vi "Register Message Metadata.vi"(8 "error in":errorcluster, 10 "Messages":T2[](array[typedef]), 11 "gRPCid in":T1) -> (0 "error out":errorcluster, 3 "gRPCid out":T1)   [LabVIEW 2019, in "grpc-lvsupport.lvlib"]
uses:
  grpc-lvsupport.lvlib
  typeDefs/Message Metadata.ctl
  typeDefs/Message Element Metadata.ctl
  typeDefs/Message Element Type.ctl
  Shared/grpcId.ctl
  <vilib>/Utility/error.llb/Error Cluster From Error Code.vi
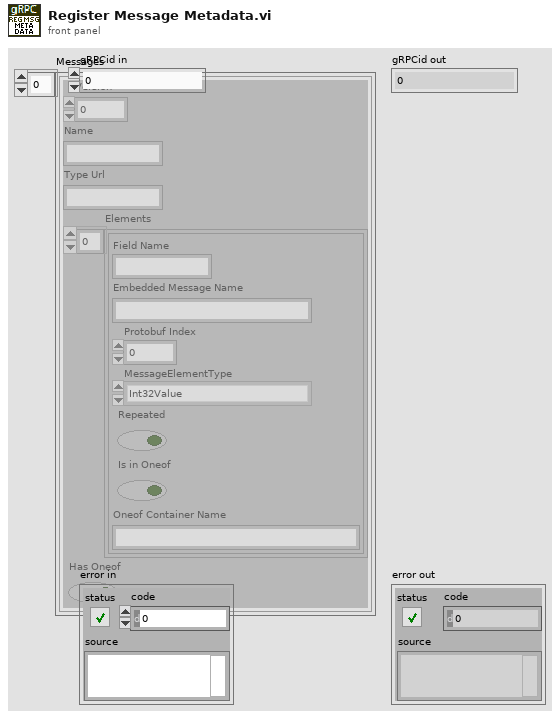
[diagram p1: front panel]
types:
  T1 = typedef "grpc-lvsupport.lvlib/grpcId.ctl" = u64
  T2 = typedef "grpc-lvsupport.lvlib/Message Metadata.ctl" = cluster{"Version":i32, "Name":string, "Type Url":string, "Elements":T3[], "Has Oneof":bool}
  T3 = typedef "grpc-lvsupport.lvlib/Message Element Metadata.ctl" = cluster{"Field Name":string, "Embedded Message Name":string, "Protobuf Index":i32, "MessageElementType":T4, "Repeated":bool, "Is in Oneof":bool, "Oneof Container Name":string}
  T4 = typedef "grpc-lvsupport.lvlib/Message Element Type.ctl" = enum32{"Int32Value", "FloatValue", "DoubleValue", "BoolValue", "StringValue", "MessageValue", "Int64Value", "UInt32Value", "UInt64Value", "EnumValue", "Bytes", "Fixed64", "Fixed32", "SFixed64", "SFixed32", "SInt64", "SInt32"}
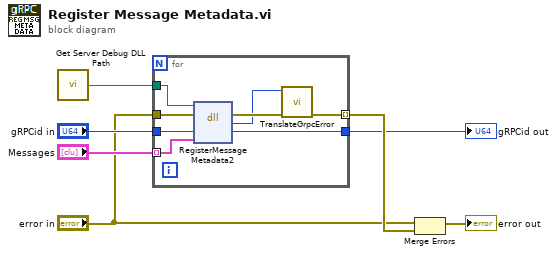
[diagram p0: block diagram]
diagram:
  n1 = call "Get Server Debug DLL Path.vi"() -> ("Server Debug DLL Path"=w3:path)
  n2 = for {
    tunnel: "Messages" -> [w13] mode=indexing
    tunnel: "gRPCid in" -> [w12]
    tunnel: "error in" -> [w15]
    tunnel: [w9] -> w7 mode=indexing
    tunnel: [w11] -> w4
    tunnel: w3 -> [w10]
    n3 = dll-call lib="?" fn="RegisterMessageMetadata2"(path in=w10, error in=w15, "serverId"=w12, "metadata"=w13) -> (error out=w14:errorcluster, "return type"=w8:i32, "serverId"=w11:T1)  [unwired: 2 in, 1 out]
    n4 = call "TranslateGrpcError.vi"("error in"=w14, "Error Code"=w8) -> ("error out"=w9:errorcluster)  [unwired: 9 in]
  }
  "gRPCid out" <- w4
  n5 = Merge Errors("error in", w7) -> (→"error out":errorcluster)
